vi "Create Message Queue.vi"(8 "error in (no error)":errorcluster) -> (0 "error out":errorcluster, 3 "Queue out":refnum<queue>)   [LabVIEW 2018]
uses:
  MessageQueueData.ctl
  Command.ctl
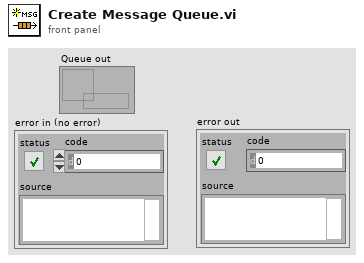
[diagram p1: front panel]
types:
  T1 = typedef "MessageQueueData.ctl" = cluster{"State":T2, "Data":variant}
  T2 = typedef "Command.ctl" = enum16{"Underbody Wash", "Soap Application", "Main High-Pressure Wash", "Clear Water Rinse", "Air Dry Cycle", "Stop"}
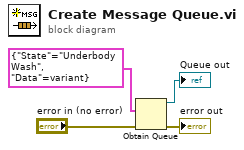
[diagram p0: block diagram]
diagram:
  n1 = Obtain Queue(element data type=T1 {"State"=enum."Underbody Wash", "Data"=variant}, error in (no error)="error in (no error)") -> (queue out=→"Queue out":refnum<queue>, error out=→"error out":errorcluster)  [unwired: 3 in, 1 out]
